vi "Main.vi"(8 "error in (no error)":errorcluster, 11 "Output Process in":refnum<class "Output Process.lvclass">) -> (0 "error out":errorcluster, 3 "Output Process out":refnum<class "Output Process.lvclass">)   [LabVIEW 2019, in "TimingDRV Engine.lvlib" / "Output Process.lvclass"]
uses:
  Output Process.lvclass
  Parent Classes/CD_Process/CD_Process.lvclass
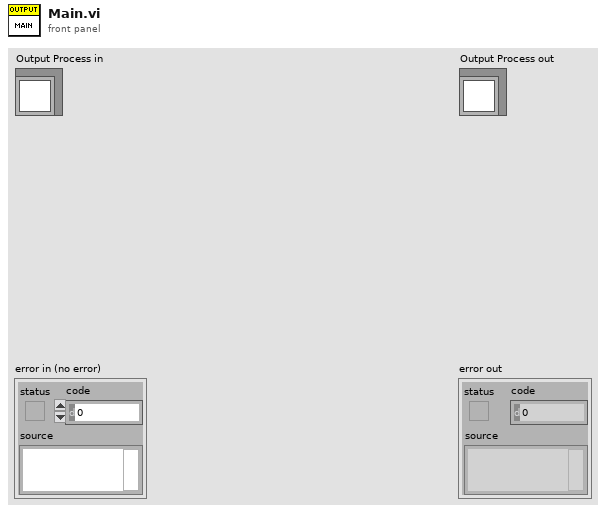
[diagram p1: front panel]
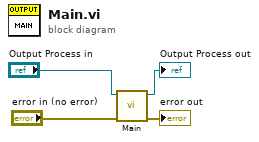
[diagram p0: block diagram]
diagram:
  n1 = call-parent "Main.vi"("error in (no error)"="error in (no error)", "CD_Process in"="Output Process in") -> ("error out"=→"error out":errorcluster, "CD_Process out"=→"Output Process out":refnum<class "Output Process.lvclass">)  [unwired: 8 in]
